vi "initializeDefaultStyle.vi"(8 "error in (no error)":errorcluster, 11 "Style in":refnum<class "Style.lvclass">) -> (0 "error out":errorcluster, 3 "Style out":refnum<class "Style.lvclass">)   [LabVIEW 2017, in "Styles.lvlib" / "Style.lvclass"]
uses:
  Style.lvclass
  Underline--ring.ctl
  Styles.lvlib
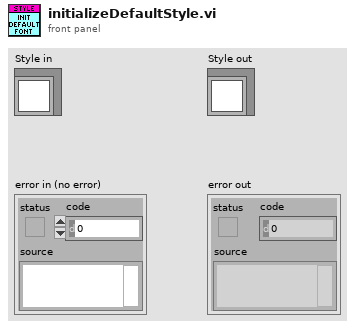
[diagram p1: front panel]
types:
  T1 = typedef "Styles.lvlib/Underline--ring.ctl" = i32
  T2 = typedef "Styles.lvlib/Font--cluster.ctl" = cluster{"Name":string, "Size":i32, "Bold":bool, "Italic":bool, "Underline":T1, "Strike":bool, "Color":u32, "Alignment":T3}
  T3 = typedef "Styles.lvlib/Alignment--ring.ctl" = i32
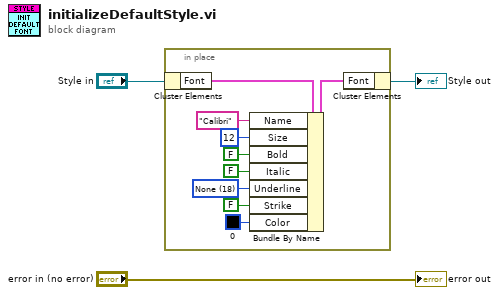
[diagram p0: block diagram]
diagram:
  n1 = in-place {
    w8 = T1 18 items=["Single"=1, "Words"=2, "Double"=3, "Thick"=4, "Dotted"=5, "DottedHeavy"=6, "Dash"=7, "DashedHeavy"=8, "DashLong"=9, "DashLongHeavy"=10, "DotDash"=11, "DashDotHeavy"=12, "DotDotDash"=13, "DashDotDotHeavy"=14, "Wave"=15, "WavyHeavy"=16, "WavyDouble"=17, "None"=18] ("Underline")
    n2 = in-place-cluster #1("Style in") -> ("Font"=w5:T2)
    n3 = Bundle By Name(cluster=w5, "Name"="Calibri", "Size"=12, "Bold"=FALSE, "Italic"=FALSE, "Underline"=w8, "Strike"=FALSE, "Color"=u32 0) -> (w4:T2)
    n4 = in-place-cluster #1("Font"=w4) -> (→"Style out":refnum<class "Style.lvclass">)
  }
  "error out" <- "error in (no error)"
